vi "Do.vi"(7 "Engine Enqueuer":refnum<class "Message Enqueuer.lvclass">, 8 "error in (no error)":errorcluster, 11 "Input in":refnum<class "Input.lvclass">) -> (0 "error out":errorcluster, 4 "Stop":bool)   [LabVIEW 2016, in "AssertEngine.lvlib" / "Input.lvclass"]
uses:
  Input.lvclass
  <vilib>/ActorFramework/Message Enqueuer/Message Enqueuer.lvclass
  Input.lvclass/Input.ctl
  AssertEngine Messages/Update Assert Data Msg/Update Assert Data Msg.lvclass/Update Assert Data Msg.ctl
  <vilib>/ActorFramework/Message Enqueuer/Message Enqueuer.lvclass/Message Enqueuer.ctl
  <vilib>/ActorFramework/Message Enqueuer/Enqueue.vi
  AssertEngine Messages/Update Assert Data Msg/Update Assert Data Msg.lvclass
  C:/Program Files/National Instruments/LabVIEW 2016/vi.lib/ActorFramework/Message/Message.lvclass
  <vilib>/ActorFramework/Message Priority Queue/Priority Enqueue.vi
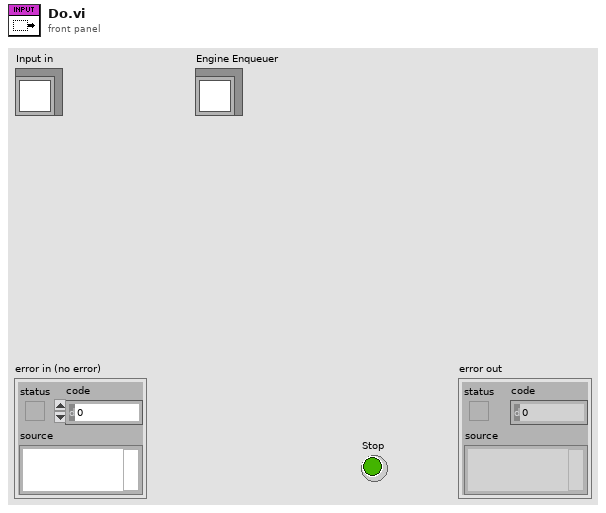
[diagram p1: front panel]
types:
  T1 = typedef "AssertEngine.lvlib/Assert Data.ctl" = cluster{"Assert Data":string, "Status":string}
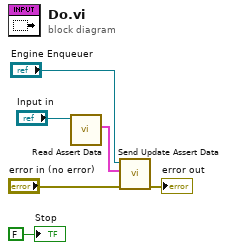
[diagram p0: block diagram]
diagram:
  n1 = call "Read Assert Data.vi"("Input in"="Input in") -> ("Assert Data"=w4:T1)  [unwired: 10 in]
  n2 = call "Send Update Assert Data.vi"("error in (no error)"="error in (no error)", "Assert Data"=w4, "Message Enqueuer"="Engine Enqueuer") -> ("error out"=→"error out":errorcluster)  [unwired: 7 in, 1 out]
  "Stop" <- FALSE ("Stop")
